vi "Array zusammenstutzen Druckregler.vi"(10 "Anzahl Elemente":i32, 11 "Daten 1":sgl[][](array[numeric])) -> (3 "Daten 1":sgl[][](array[numeric]))   [LabVIEW 2020, in "Erweiterte Konfig.lvlib"]
uses:
  Erweiterte Konfig.lvlib
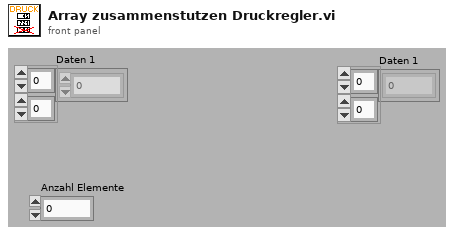
[diagram p1: front panel]
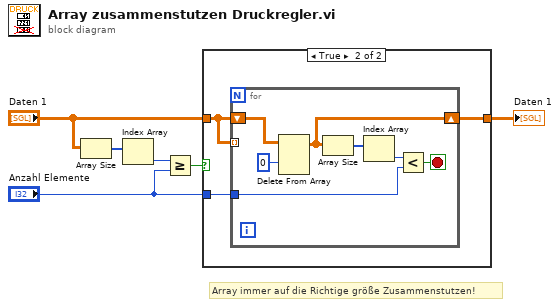
[diagram p0: block diagram]
diagram:
  # "Array immer auf die Richtige größe Zusammenstutzen!"
  n1 = Array Size(array="Daten 1") -> (size(s)=w4:i32[])
  n2 = Index Array(array=w4) -> (element=w3:i32)  [unwired: 1 in]
  n3 = Greater Or Equal?(x=w3, y="Anzahl Elemente") -> (x >= y?=w6:bool)
  n4 = case shown="True" w6 {
    tunnel: "Daten 1" -> [w7 w9]
    tunnel: [w7 w8] -> w2
    tunnel: "Anzahl Elemente" -> [_ w10]
    frame False {
    }
    frame True {
      n5 = for {
        tunnel: w10 -> [w16]
        tunnel: w9 -> [_] mode=indexing
        shift-right: [w13] -> w8
        shift-left: w9 -> [w17]
        stop <- w15 stop-if-true
        n6 = Delete From Array(array=w17, index (row)=0 ("Index")) -> (array with subset deleted=w13:sgl[][])  [unwired: 2 in, 1 out]
        n7 = Array Size(array=w13) -> (size(s)=w12:i32[])
        n8 = Index Array(array=w12) -> (element=w11:i32)  [unwired: 1 in]
        n9 = Less?(x=w11, y=w16) -> (x < y?=w15:bool)
      }
    }
  }
  "Daten 1" <- w2
